vi "generate arrays for pockels cell blanking.vi"() -> (3 "Array":dbl[][](array[numeric]))   [LabVIEW 2012]
doc: "SciScan 1.0 151216"
uses:
  Custom Controls/biotfile select.ctl
  GFG/GFGbooleanGet.vi
  GFG/GFGnumericGet.vi
  GFG/GFG library.lvlib
panel:
  out "number of pockels cell ao samples per line":dbl=65.0
  in  "n":i32
  out "size(s)":i32
  out "piezo data":dbl[](graph)
  out "pockels blanking data":dbl[](graph)
  in  "min pockels cell voltage":dbl
  out "number of pcao samples to blank on each side":dbl
  out "example piezo array":dbl[](graph)
  out "example pockels cell data":dbl[](graph)
  out "Waveform Graph":dbl[][](graph)
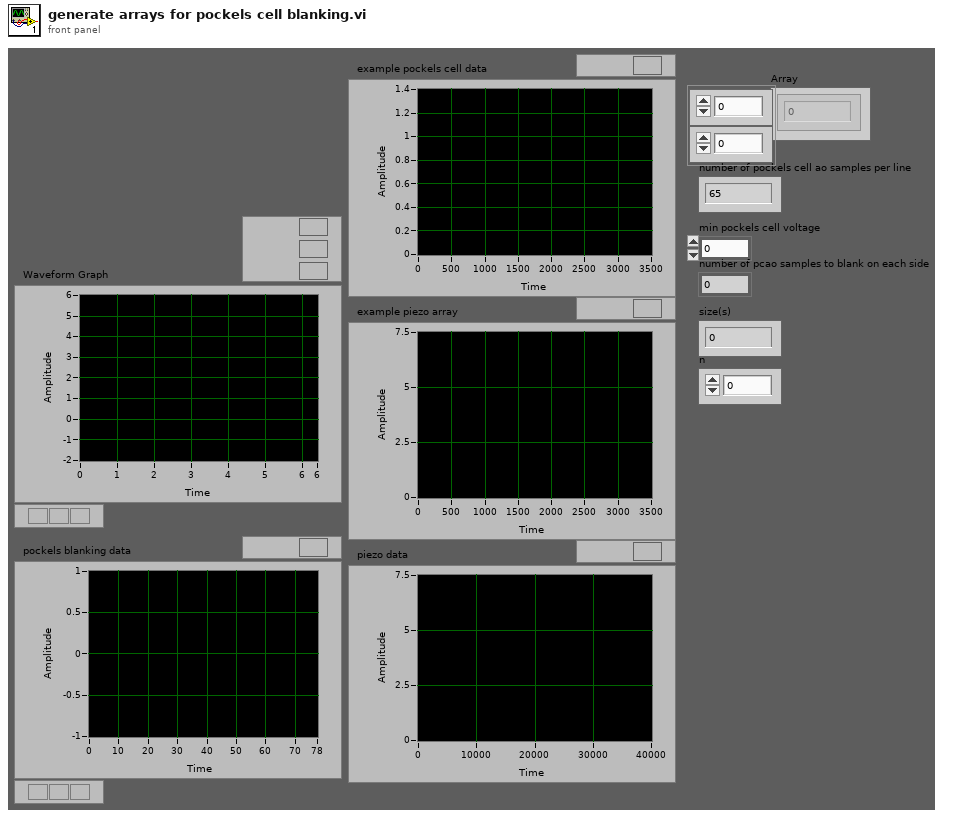
[diagram p1: front panel]
types:
  T1 = typedef "biotfile select.ctl" = enum16{"7962with5751_512px_40Mhz", "7962with5751_512px_50Mhz", "7961with5734_1024px_120Mhz or ext lasersync", "7962with5734_1024px_120Mhz or ext lasersync", "7962with5734_512px_120Mhz or ext lasersync", "7961with5734_512px_120Mhz or ext lasersync", "7962with5751_12kHz_512px_50MHz_4ch", "7962with5751_1536px_2ch_40Mhz", "7962with5751_1536px_2ch_50Mhz", "7962with5751_12kHz_1024px_2ch_50MHz"}
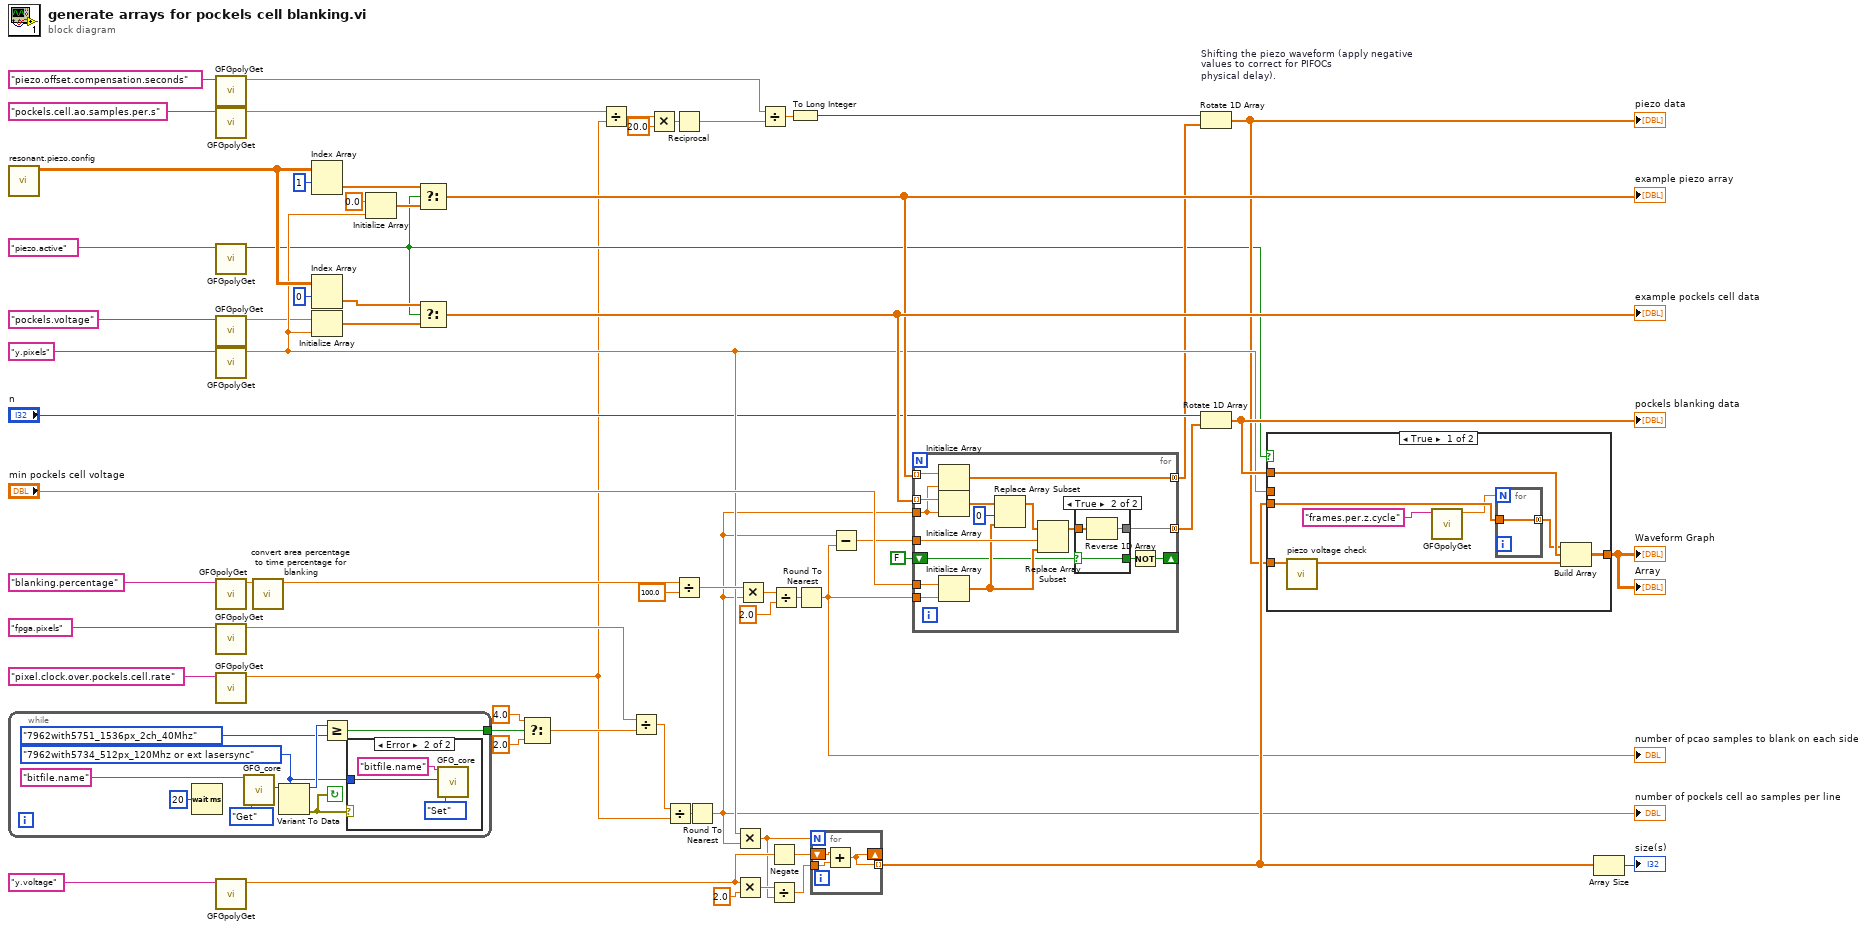
[diagram p0: block diagram]
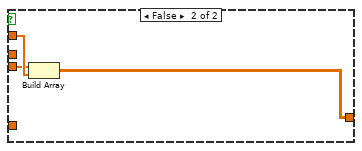
[diagram p4: hidden frame]
diagram:
  n1 = call "resonant.piezo.config.vi"() -> ("appended array"=w57:dbl[][])  [unwired: 11 in]
  n2 = while {
    tunnel: [w68] -> w27
    stop <- w66 continue-if-true
    w65 = biotfile_select."7962with5734_512px_120Mhz or ext lasersync" ("bitfile name")
    n3 = Wait (ms)(milliseconds to wait=u32 20) -> ()  [unwired: 1 out]
    n4 = call "GFG_core.vi"("Variable Name in"="bitfile.name", "Action"=enum16{"Init", "Set", "Get", "Clear"}."Get") -> ("Variant Out"=w71:variant)  [unwired: 11 in, 6 out]
    n5 = Variant To Data(type=w65, Variant=w71) -> (data=w70:T1, error out=w66:errorcluster)  [unwired: 1 in]
    n6 = Greater Or Equal?(x=w70, y=biotfile_select."7962with5751_1536px_2ch_40Mhz" ("bitfile name")) -> (x >= y?=w68:bool)
    n7 = case shown="Error" w66 {
      tunnel: w65 -> [_ w74]
      frame No Error {
      }
      frame Error {
        n8 = call "GFG_core.vi"("Variable Name in"="bitfile.name", "Variant in"=w74, "Action"=enum16{"Init", "Set", "Get", "Clear"}."Set") -> ()  [unwired: 10 in, 7 out]
      }
    }
  }
  n9 = call-poly "GFGpolyGet.vi"("Variable Name in"="piezo.offset.compensation.seconds") -> ("Numeric"=w15:dbl)  [unwired: 8 in, 2 out]
  n10 = call-poly "GFGpolyGet.vi"("Variable Name in"="pockels.cell.ao.samples.per.s") -> ("Numeric"=w11:dbl)  [unwired: 8 in, 2 out]
  n11 = call-poly "GFGpolyGet.vi"("Variable Name in"="piezo.active") -> ("Boolean Value OUT"=w8:bool)  [unwired: 9 in, 1 out]
  n12 = call-poly "GFGpolyGet.vi"("Variable Name in"="pockels.voltage") -> ("Numeric"=w36:dbl)  [unwired: 8 in, 2 out]
  n13 = call-poly "GFGpolyGet.vi"("Variable Name in"="y.pixels") -> ("Numeric"=w44:dbl)  [unwired: 8 in, 2 out]
  n14 = call-poly "GFGpolyGet.vi"("Variable Name in"="blanking.percentage") -> ("Numeric"=w31:dbl)  [unwired: 8 in, 2 out]
  n15 = call-poly "GFGpolyGet.vi"("Variable Name in"="fpga.pixels") -> ("Numeric"=w34:dbl)  [unwired: 8 in, 2 out]
  n16 = call-poly "GFGpolyGet.vi"("Variable Name in"="pixel.clock.over.pockels.cell.rate") -> ("Numeric"=w1:dbl)  [unwired: 8 in, 2 out]
  n17 = call-poly "GFGpolyGet.vi"("Variable Name in"="y.voltage" ("Tag in")) -> ("Numeric"=w38:dbl)  [unwired: 8 in, 2 out]
  n18 = call "convert area percentage to time percentage for blanking.vi"("areapercentage"=w31) -> ("timepercentage"=w30:dbl)  [unwired: 10 in]
  n19 = Index Array(array=w57, index (row)=1 ("index")) -> (element=w47:dbl[])  [unwired: 1 in]
  n20 = Index Array(array=w57, index (row)=0 ("index")) -> (element=w49:dbl[])  [unwired: 1 in]
  n21 = Initialize Array(w36, w44) -> (w45:dbl[])
  n22 = Initialize Array(0.0 ("element"), w44) -> (w42:dbl[])
  n23 = Select(t=w47, s=w8, f=w42) -> (s? t:f=w46:dbl[])
  "example piezo array" <- w46
  n24 = Select(t=w49, s=w8, f=w45) -> (s? t:f=w48:dbl[])
  "example pockels cell data" <- w48
  n25 = Select(t=4.0 ("y"), s=w27, f=2.0 ("y")) -> (s? t:f=w26:dbl)
  n26 = Divide(x=w11, y=w1) -> (x/y=w10:dbl)
  n27 = Divide(x=w34, y=w26) -> (x/y=w53:dbl)
  n28 = Multiply(x=w10, y=20.0) -> (x*y=w21:dbl)
  n29 = Divide(x=w53, y=w1) -> (x/y=w32:dbl)
  n30 = Reciprocal(x=w21) -> (1/x=w16:dbl)
  n31 = Divide(x=w30, y=100.0) -> (x/y=w62:dbl)
  n32 = Round To Nearest(number=w32) -> (nearest integer value=w41:dbl)
  "number of pockels cell ao samples per line" <- w41
  n33 = Multiply(x=w44, y=w41) -> (x*y=w3:dbl)
  n34 = Multiply(x=w38, y=2.0) -> (x*y=w6:dbl)
  n35 = Multiply(x=w62, y=w41) -> (x*y=w61:dbl)
  n36 = Divide(x=w15, y=w16) -> (x/y=w19:dbl)
  n37 = Negate(x=w38) -> (-x=w5:dbl)
  n38 = Divide(x=w6, y=w3) -> (x/y=w4:dbl)
  n39 = Divide(x=w61, y=2.0 ("x")) -> (x/y=w23:dbl)
  n40 = To Long Integer(number=w19) -> (32bit integer=w18:i32)
  n41 = Round To Nearest(number=w23) -> (nearest integer value=w51:dbl)
  "number of pcao samples to blank on each side" <- w51
  n42 = for {
    N: w3 -> [_]
    tunnel: w4 -> [w78]
    shift-right: [w77] -> _
    shift-left: w5 -> [w79]
    tunnel: [w77] -> w56 mode=indexing
    n43 = Add(x=w79, y=w78) -> (x+y=w77:dbl)
  }
  n44 = Subtract(x=w41, y=w51) -> (x-y=w22:dbl)
  n45 = for {
    tunnel: w48 -> [w95] mode=indexing
    tunnel: w41 -> [w89]
    tunnel: w22 -> [w93]
    tunnel: [w83] -> w17 mode=concatenating
    tunnel: w51 -> [w92]
    tunnel: "min pockels cell voltage" -> [w91]
    tunnel: w46 -> [w90] mode=indexing
    tunnel: [w87] -> w14 mode=concatenating
    shift-right: [w81] -> _
    shift-left: FALSE -> [w82]
    n46 = Initialize Array(w90, w89) -> (w87:dbl[])
    n47 = Initialize Array(w95, w89) -> (w86:dbl[])
    n48 = Initialize Array(w91, w92) -> (w88:dbl[])
    n49 = Replace Array Subset(array=w86, new element=w88, index=0) -> (w85:dbl[])
    n50 = Replace Array Subset(array=w85, new element=w88, index=w93) -> (w84:dbl[])
    n51 = case shown="True" w82 {
      selector: w82 -> [w96 w98]
      tunnel: w84 -> [w97 w100]
      tunnel: [w97 w99] -> w83
      tunnel: [w96 w98] -> w80
      frame False {
      }
      frame True {
        n52 = Reverse 1D Array(array=w100) -> (reversed array=w99:dbl[])
      }
    }
    n53 = Not(x=w80) -> (.not. x?=w81:bool)
  }
  n54 = Rotate 1D Array "Shifting the piezo waveform (apply negative values to correct for PIFOCs\nphysical delay)."(1:w14, 2:w18) -> (0:w13:dbl[])
  "piezo data" <- w13
  n55 = Rotate 1D Array(1:w17, 2:"n") -> (0:w50:dbl[])
  "pockels blanking data" <- w50
  n56 = case shown="True" w8 {
    tunnel: w56 -> [w107 w110]
    tunnel: w44 -> [_ _]
    tunnel: [w104 w111] -> w2
    tunnel: w50 -> [w106 w112]
    tunnel: w13 -> [w102 _]
    frame True {
      n57 = call "piezo voltage check.vi"("piezo array in"=w102) -> ("piezo array out"=w101:dbl[])  [unwired: 10 in]
      n58 = call-poly "GFGpolyGet.vi"("Variable Name in"="frames.per.z.cycle" ("Tag in")) -> ("Numeric"=w103:dbl)  [unwired: 8 in, 2 out]
      n59 = for {
        N: w103 -> [_]
        tunnel: w107 -> [w109]
        tunnel: [w109] -> w105 mode=concatenating
      }
      n60 = Build Array(w105, w106, w101) -> (w104:dbl[][])
    }
    frame False {
      n61 = Build Array(w110, w112) -> (w111:dbl[][])
    }
  }
  "Array" <- w2
  "Waveform Graph" <- w2
  n62 = Array Size(array=w56) -> (size(s)=→"size(s)":i32)
